vi "2D Random Walk Exercise - Gavin Branyon (1).vi"() -> ()   [LabVIEW 2019]
uses:
  <vilib>/numeric/Random Number (Range) I64.vi
  <vilib>/numeric/sub_Random U32.vi
panel:
  out "XY Graph":cluster{"number":i64, "number":i64}[](graph)
  # "Gavin Branyon\n2/12/2024\n2D Random Walk Exercise"
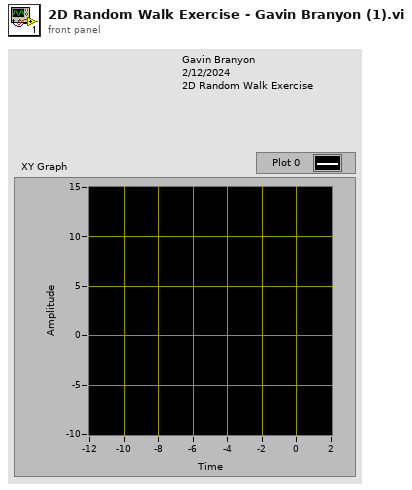
[diagram p1: front panel]
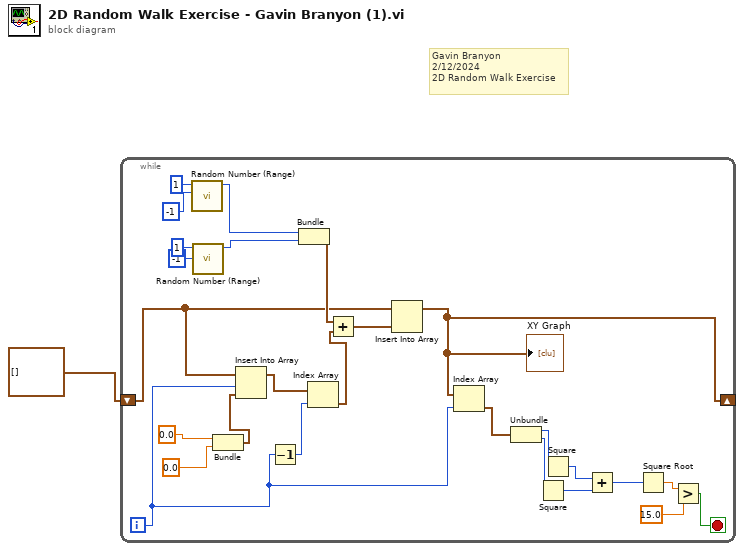
[diagram p0: block diagram]
diagram:
  # "Gavin Branyon\n2/12/2024\n2D Random Walk Exercise"
  n1 = while {
    shift-right: [w3] -> _
    shift-left: cluster{"number":i64, "number":i64}[] [] ("output array") -> [w19]
    i -> [w13]
    stop <- w4 stop-if-true
    n2 = call-poly <vilib>:"Random Number (Range).vi"("lower bound (-100)"=i64 -1, "upper bound (100)"=i64 1) -> ("number"=w23:i64)  [unwired: 9 in]
    n3 = call-poly <vilib>:"Random Number (Range).vi"("lower bound (-100)"=i64 -1, "upper bound (100)"=i64 1) -> ("number"=w22:i64)  [unwired: 9 in]
    n4 = Bundle(0.0, 0.0) -> (w16:cluster{dbl, dbl})  [unwired: 1 in]
    n5 = Insert Into Array(array=w19, index=w13, new element=w16) -> (w15:cluster{"number":i64, "number":i64}[])
    n6 = Decrement(x=w13) -> (x-1=w14:i32)
    n7 = Bundle("number"=w23, "number"=w22) -> (w20:cluster{"number":i64, "number":i64})  [unwired: 1 in]
    n8 = Index Array(array=w15, index=w14) -> (element=w2:cluster{"number":i64, "number":i64})
    n9 = Add(x=w20, y=w2) -> (x+y=w21:cluster{"number":i64, "number":i64})
    n10 = Insert Into Array(array=w19, new element=w21) -> (w3:cluster{"number":i64, "number":i64}[])  [unwired: 1 in]
    "XY Graph" <- w3
    n11 = Index Array(array=w3, index=w13) -> (element=w12:cluster{"number":i64, "number":i64})
    n12 = Unbundle(w12) -> ("number"=w11:i64, "number"=w10:i64)
    n13 = Square(x=w10) -> (x^2=w8:i64)
    n14 = Square(x=w11) -> (x^2=w9:i64)
    n15 = Add(x=w9, y=w8) -> (x+y=w7:i64)
    n16 = Square Root(x=w7) -> (sqrt(x)=w5:dbl)
    n17 = Greater?(x=w5, y=15.0) -> (0:w4:bool)
  }
